vi "Add Icon From Image Data.vi"(7 "Icon Index (Next)":i32=-1, 8 "error in (no error)":errorcluster, 9 "Icon Name":string, 10 "Image Data":T1, 11 "Toolbar Control in":refnum<class "Toolbar Control.lvclass">) -> (0 "error out":errorcluster, 3 "Toolbar Control out":refnum<class "Toolbar Control.lvclass">)   [LabVIEW 2011, in "Toolbar Control.lvclass"]
doc: "This VI will add the image <B>Image Data</B> to the <B>Toolbar Control in</B> at the available location or if specified by <B>Icon Index (Next)</B>. The name of the icon is specified by <B>Icon Name</B>.\n\n-------------\nDeveloped by Brian Hoover (hooovahh)"
uses:
  Toolbar Control.lvclass
  <vilib>/picture/picture.llb/imagedata.ctl
  Toolbar Control.lvclass/Toolbar Control.ctl
  Controls/Icon Data.ctl
  Controls/Button State.ctl
  Controls/Icon Type.ctl
  <vilib>/Utility/miscctls.llb/LVRectTypeDef.ctl
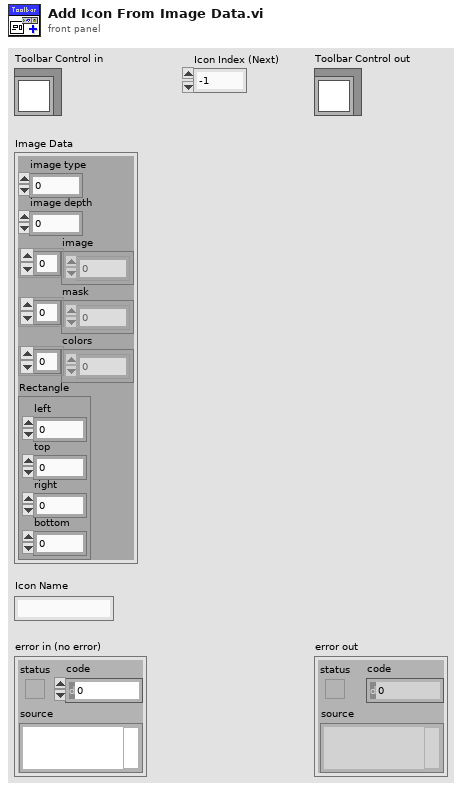
[diagram p1: front panel]
types:
  T1 = typedef "imagedata.ctl" = cluster{"image type":i32, "image depth":i32, "image":u8[], "mask":u8[], "colors":u32[], "Rectangle":cluster{"left":i16, "top":i16, "right":i16, "bottom":i16}}
  T2 = typedef "LVRectTypeDef.ctl" = cluster{"Left":i16, "Top":i16, "Right":i16, "Bottom":i16}
  T3 = typedef "Toolbar Control.lvclass/Icon Data.ctl" = cluster{"Original Image Path":path, "Original Image Data":T1, "Scaled Icon":picture, "Button Name":string, "Button State":T4, "Icon Type":T5}
  T4 = typedef "Toolbar Control.lvclass/Button State.ctl" = enum8{"Enabled", "Disabled", "Disabled and Grayed Out"}
  T5 = typedef "Icon Type.ctl" = enum16{"Normal Icon", "Separator Icon", "More Options"}
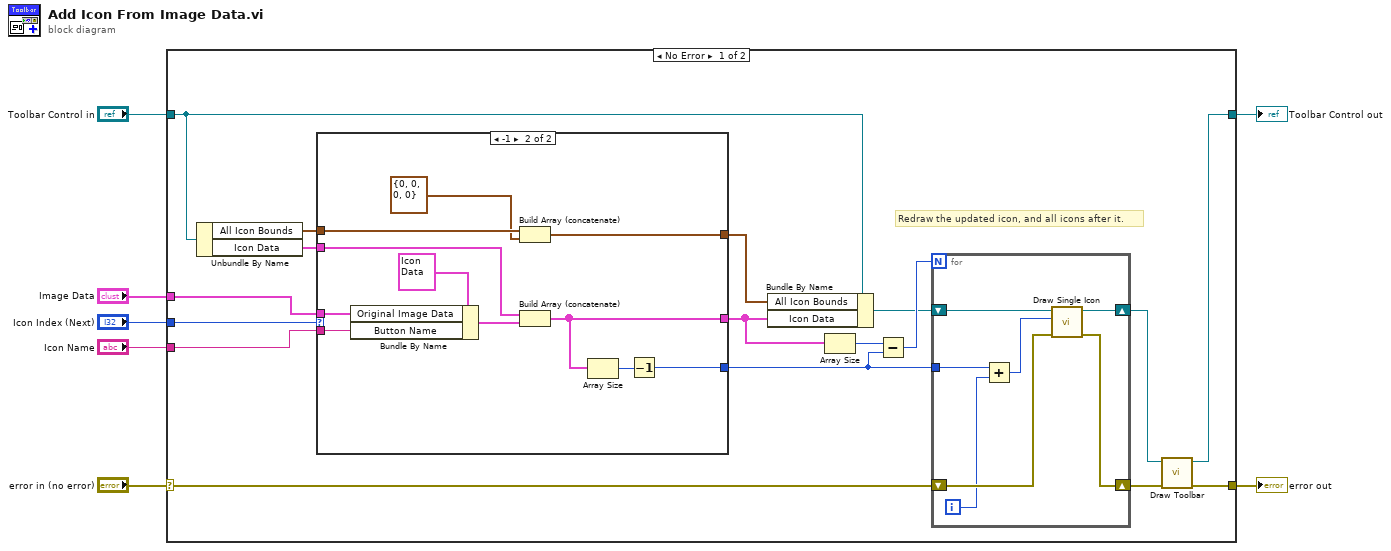
[diagram p0: block diagram]
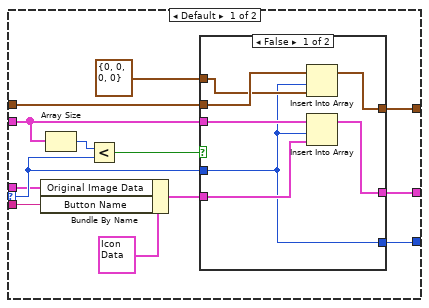
[diagram p2: hidden frame]
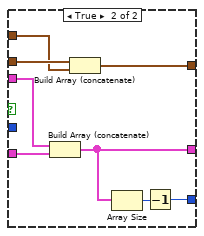
[diagram p3: hidden frame]
diagram:
  n1 = case shown="No Error" "error in (no error)" {
    selector: "error in (no error)" -> [w12 w72]
    tunnel: [w8 w72] -> w6
    tunnel: [w9 w71] -> w4
    tunnel: "Toolbar Control in" -> [w24 w71]
    tunnel: "Image Data" -> [w22 _]
    tunnel: "Icon Index (Next)" -> [w21 _]
    tunnel: "Icon Name" -> [w20 _]
    frame No Error {
      # "Redraw the updated icon, and all icons after it."
      n2 = Unbundle By Name(w24) -> ("All Icon Bounds"=w19:T2[], "Icon Data"=w23:T3[])
      n3 = case shown="-1" w21 {
        selector: w21 -> [w37 _]
        tunnel: w22 -> [w36 w69]
        tunnel: w20 -> [w44 w68]
        tunnel: w23 -> [w42 w67]
        tunnel: [w38 w64] -> w14
        tunnel: [w35 w63] -> w15
        tunnel: w19 -> [w34 w62]
        tunnel: [w33 w61] -> w18
        frame Default {
          n4 = Bundle By Name(cluster=T3 {"Original Image Path"=path "", "Original Image Data"={"image type"=0, "image depth"=0, "image"=[], "mask"=[], "colors"=[], "Rectangle"={"left"=0, "top"=0, "right"=0, "bottom"=0}}, "Scaled Icon"=bytes[0], "Button Name"="", "Button State"=enum."Enabled", "Icon Type"=enum."Normal Icon"} ("Cluster"), "Original Image Data"=w36, "Button Name"=w44) -> (w39:T3)
          n5 = Array Size(array=w42) -> (size(s)=w41:i32)
          n6 = Less?(x=w41, y=w37) -> (x < y?=w40:bool)
          n7 = case shown="False" w40 {
            tunnel: w42 -> [w51 w59]
            tunnel: w39 -> [w50 w58]
            tunnel: [w49 w55] -> w38
            tunnel: w37 -> [w45 _]
            tunnel: [w45 w56] -> w35
            tunnel: w34 -> [w47 w54]
            tunnel: [w48 w53] -> w33
            tunnel: T2 {"Left"=0, "Top"=0, "Right"=0, "Bottom"=0} ("Icon Bounds") -> [w46 w52]
            frame False {
              n8 = Insert Into Array(array=w47, index=w45, new element=w46) -> (w48:T2[])
              n9 = Insert Into Array(array=w51, index=w45, new element=w50) -> (w49:T3[])
            }
            frame True {
              n10 = Build Array (concatenate)(w59, w58) -> (w55:T3[])
              n11 = Build Array (concatenate)(w54, w52) -> (w53:T2[])
              n12 = Array Size(array=w55) -> (size(s)=w57:i32)
              n13 = Decrement(x=w57) -> (x-1=w56:i32)
            }
          }
        }
        frame -1 {
          n14 = Bundle By Name(cluster=T3 {"Original Image Path"=path "", "Original Image Data"={"image type"=0, "image depth"=0, "image"=[], "mask"=[], "colors"=[], "Rectangle"={"left"=0, "top"=0, "right"=0, "bottom"=0}}, "Scaled Icon"=bytes[0], "Button Name"="", "Button State"=enum."Enabled", "Icon Type"=enum."Normal Icon"} ("Cluster"), "Original Image Data"=w69, "Button Name"=w68) -> (w66:T3)
          n15 = Build Array (concatenate)(w62, T2 {"Left"=0, "Top"=0, "Right"=0, "Bottom"=0} ("Icon Bounds")) -> (w61:T2[])
          n16 = Build Array (concatenate)(w67, w66) -> (w64:T3[])
          n17 = Array Size(array=w64) -> (size(s)=w65:i32)
          n18 = Decrement(x=w65) -> (x-1=w63:i32)
        }
      }
      n19 = Bundle By Name(cluster=w24, "All Icon Bounds"=w18, "Icon Data"=w14) -> (w13:refnum<class "Toolbar Control.lvclass">)
      n20 = Array Size(array=w14) -> (size(s)=w17:i32)
      n21 = Subtract(x=w17, y=w15) -> (x-y=w16:i32)
      n22 = for {
        N: w16 -> [_]
        tunnel: w15 -> [w27]
        shift-right: [w30] -> w10
        shift-left: w13 -> [w31]
        shift-right: [w28] -> w11
        shift-left: w12 -> [w29]
        i -> [w26]
        n23 = Add(x=w27, y=w26) -> (x+y=w25:i32)
        n24 = call "Draw Single Icon.vi"("error in (no error)"=w29, "Icon Index"=w25, "Toolbar Control in"=w31) -> ("error out"=w28:errorcluster, "Toolbar Control out"=w30:refnum<class "Toolbar Control.lvclass">)  [unwired: 7 in]
      }
      n25 = call "Draw Toolbar.vi"("error in (no error)"=w11, "Toolbar Control in"=w10) -> ("error out"=w8:errorcluster, "Toolbar Control out"=w9:refnum<class "Toolbar Control.lvclass">)  [unwired: 7 in, 1 out]
    }
    frame Error {
    }
  }
  "error out" <- w6
  "Toolbar Control out" <- w4
